vi "Get.vi"(0 "InfluxDB Client in":refnum<class "Client.lvclass">, 5 "Query":T1, 11 "error in (no error)":errorcluster) -> (4 "InfluxDB Client out":refnum<class "Client.lvclass">, 6 "body":string, 8 "Status code":string, 10 "Headers":T1, 15 "error out":errorcluster)   [LabVIEW 2018, in "InfluxDB Client.lvlib" / "Client.lvclass"]
uses:
  Client.lvclass
  <userlib>/_OpenG.lib/dictionary/dictionary.llb/Dictionary Object RefNum__ogtk.ctl
  <userlib>/_OpenG.lib/dictionary/dictionary.llb/Dictionary Object RefNum - Enum__ogtk.ctl
  Client.lvclass/Client.ctl
  <vilib>/httpClient/POSTBuffer.vi
  <vilib>/httpClient/LabVIEWHTTPClient.lvlib
panel:
  out "query":string
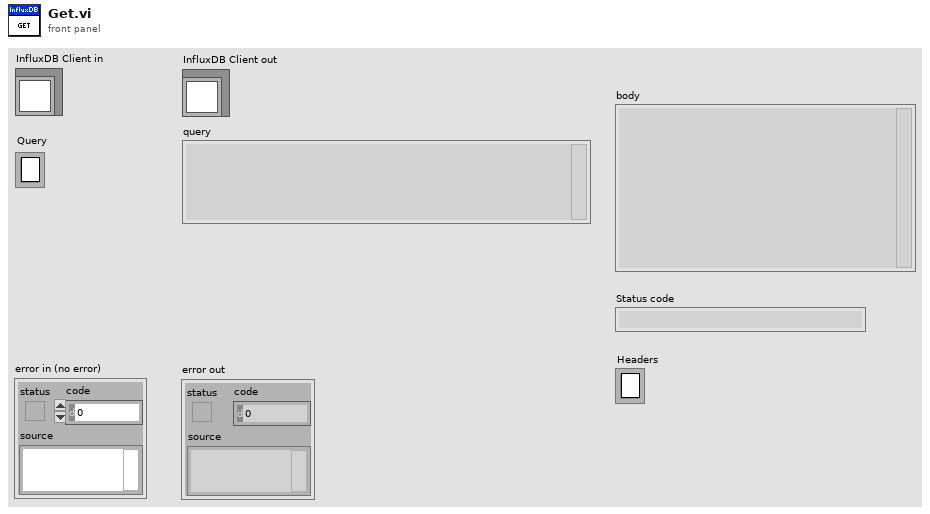
[diagram p1: front panel]
types:
  T1 = typedef "Dictionary Object RefNum__ogtk.ctl" = refnum<k1>
  T2 = typedef "LabVIEWHTTPClient.lvlib/ClientHandle.ctl" = refnum<k1>
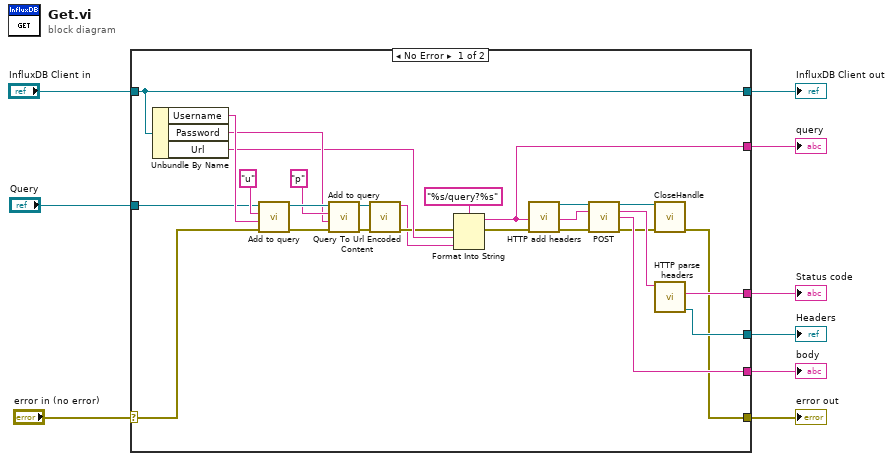
[diagram p0: block diagram]
diagram:
  n1 = case shown="No Error" "error in (no error)" {
    selector: "error in (no error)" -> [w17 w37]
    tunnel: [w10 w37] -> w8
    tunnel: [w35 w36] -> w6
    tunnel: "InfluxDB Client in" -> [w35 w36]
    tunnel: "Query" -> [w21 _]
    tunnel: [w15 _] -> w4
    tunnel: [w14 _] -> w3
    tunnel: [w13 _] -> w2
    tunnel: [w12 _] -> w1
    frame No Error {
      n2 = Unbundle By Name(w35) -> ("Username"=w33:string, "Password"=w30:string, "Url"=w23:string)
      n3 = call "Add to query.vi"("error in (no error)"=w17, "Value"=w33, "Parameter"="u", "Query in"=w21) -> ("error out"=w20:errorcluster, "Query out"=w32:T1)  [unwired: 6 in]
      n4 = call "Add to query.vi"("error in (no error)"=w20, "Value"=w30, "Parameter"="p", "Query in"=w32) -> ("error out"=w19:errorcluster, "Query out"=w22:T1)  [unwired: 6 in]
      n5 = call "Query To Url Encoded Content.vi"("error in (no error)"=w19, "Query"=w22) -> ("error out"=w18:errorcluster, "Url Encoded Content"=w16:string)  [unwired: 8 in]
      n6 = Format Into String(format string="%s/query?%s", error in=w18, w23, w16) -> (resulting string=w15:string, error out=w24:errorcluster)  [unwired: 1 in]
      n7 = call "HTTP add headers.vi"("error in (no error)"=w24) -> ("client handle out"=w26:T2, "error out"=w25:errorcluster)  [unwired: 13 in]
      n8 = call-poly <vilib>:"POST.vi"("client handle"=w26, "url"=w15, "error in (no error)"=w25) -> ("client handle out"=w28:T2, "headers"=w27:string, "body"=w14:string, "error out"=w11:errorcluster)  [unwired: 9 in]
      n9 = call <vilib>:"CloseHandle.vi"("client handle"=w28, "error in (no error)"=w11) -> ("error out"=w10:errorcluster)  [unwired: 13 in]
      n10 = call "HTTP parse headers.vi"("HTTP headers"=w27) -> ("Headers out"=w12:T1, "Status code"=w13:string)  [unwired: 7 in, 2 out]
    }
    frame Error {
    }
  }
  "error out" <- w8
  "InfluxDB Client out" <- w6
  "query" <- w4
  "body" <- w3
  "Status code" <- w2
  "Headers" <- w1
